vi "rx_ceEq.vi"(2 "preamble":cdb[](array[numeric])=[-0.7071067811865475+0.7071067811865476i, 0.7071067811865476+0.7071067811865475i, 0.7071067811865474-0.7071067811865477i, 0.7071067811865476+0.7071067811865475i, -0.7071067811865475+0.7071067811865476i, -0.7071067811865477-0.7071067811865475i, 0.7071067811865476+0.7071067811865475i, -0.7071067811865477-0.7071067811865475i, -0.7071067811865475+0.7071067811865476i, 0.7071067811865476+0.7071067811865475i, 0.7071067811865474-0.7071067811865477i, 0.7071067811865476+0.7071067811865475i, -0.7071067811865475+0.7071067811865476i, -0.7071067811865477-0.7071067811865475i, 0.7071067811865476+0.7071067811865475i, -0.7071067811865477-0.7071067811865475i, -0.7071067811865475+0.7071067811865476i, 0.7071067811865476+0.7071067811865475i, 0.7071067811865474-0.7071067811865477i, 0.7071067811865476+0.7071067811865475i, -0.7071067811865475+0.7071067811865476i, -0.7071067811865477-0.7071067811865475i, 0.7071067811865476+0.7071067811865475i, -0.7071067811865477-0.7071067811865475i, -0.7071067811865475+0.7071067811865476i, 0.7071067811865476+0.7071067811865475i, 0.7071067811865474-0.7071067811865477i, 0.7071067811865476+0.7071067811865475i, -0.7071067811865475+0.7071067811865476i, -0.7071067811865477-0.7071067811865475i, 0.7071067811865476+0.7071067811865475i, -0.7071067811865477-0.7071067811865475i, -0.7071067811865475+0.7071067811865476i, 0.7071067811865476+0.7071067811865475i, 0.7071067811865474-0.7071067811865477i, 0.7071067811865476+0.7071067811865475i, -0.7071067811865475+0.7071067811865476i, -0.7071067811865477-0.7071067811865475i, 0.7071067811865476+0.7071067811865475i, -0.7071067811865477-0.7071067811865475i, -0.7071067811865475+0.7071067811865476i, 0.7071067811865476+0.7071067811865475i, 0.7071067811865474-0.7071067811865477i, 0.7071067811865476+0.7071067811865475i, -0.7071067811865475+0.7071067811865476i, -0.7071067811865477-0.7071067811865475i, 0.7071067811865476+0.7071067811865475i, -0.7071067811865477-0.7071067811865475i, -0.7071067811865475+0.7071067811865476i, 0.7071067811865476+0.7071067811865475i, 0.7071067811865474-0.7071067811865477i, 0.7071067811865476+0.7071067811865475i, -0.7071067811865475+0.7071067811865476i, -0.7071067811865477-0.7071067811865475i, 0.7071067811865476+0.7071067811865475i, -0.7071067811865477-0.7071067811865475i, -0.7071067811865475+0.7071067811865476i, 0.7071067811865476+0.7071067811865475i, 0.7071067811865474-0.7071067811865477i, 0.7071067811865476+0.7071067811865475i, -0.7071067811865475+0.7071067811865476i, -0.7071067811865477-0.7071067811865475i, 0.7071067811865476+0.7071067811865475i, -0.7071067811865477-0.7071067811865475i], 3 "symbols":cdb[](array[numeric])) -> (0 "valid?":bool, 1 "eq symbols":cdb[](array[numeric]))   [LabVIEW 2014]
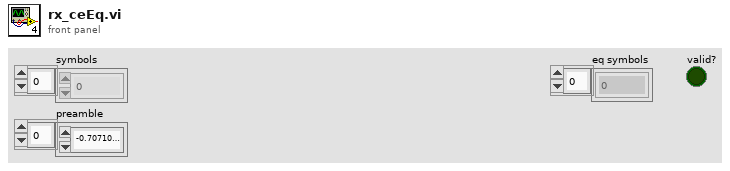
[diagram p1: front panel]
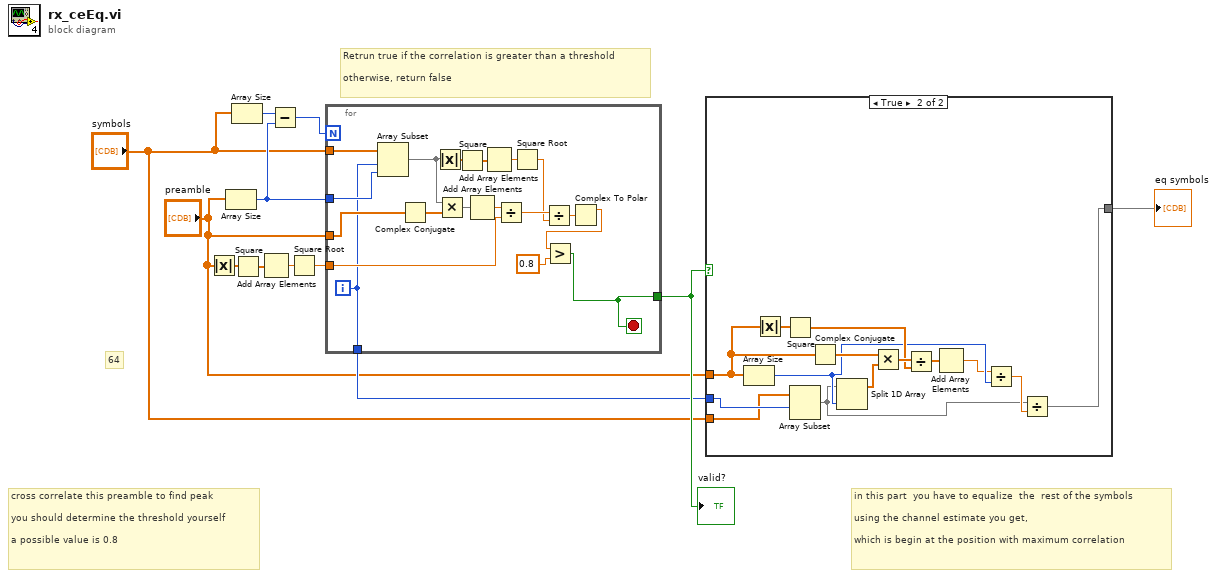
[diagram p0: block diagram]
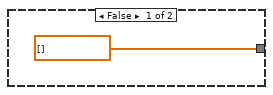
[diagram p2: hidden frame]
diagram:
  # "in this part  you have to equalize  the  rest of the symbols\n\nusing the channel estimate you get, \n\nwhich is begin at the position with maximum correlation"
  # "Retrun true if the correlation is greater than a threshold\n\notherwise, return false"
  # "cross correlate this preamble to find peak \n\nyou should determine the threshold yourself\n\na possible value is 0.8"
  # "64"
  n1 = Absolute Value(x="preamble") -> (abs(x)=w8:dbl[])
  n2 = Array Size(array="preamble") -> (size(s)=w5:i32)
  n3 = Array Size(array="symbols") -> (size(s)=w6:i32)
  n4 = Square(x=w8) -> (x^2=w11:dbl[])
  n5 = Add Array Elements(numeric array=w11) -> (sum=w10:dbl)
  n6 = Subtract(x=w6, y=w5) -> (x-y=w4:i32)
  n7 = Square Root(x=w10) -> (sqrt(x)=w9:dbl)
  n8 = for {
    N: w4 -> [_]
    tunnel: "symbols" -> [w30]
    tunnel: w5 -> [w29]
    tunnel: "preamble" -> [w23]
    tunnel: w9 -> [w21]
    tunnel: [w13] -> w7
    tunnel: [w14] -> w3
    i -> [w14]
    stop <- w13 stop-if-true
    n9 = Array Subset(array=w30, index=w14, length=w29) -> (w25:cdb[])
    n10 = Complex Conjugate(1:w23) -> (0:w24:cdb[])
    n11 = Absolute Value(x=w25) -> (abs(x)=w17:dbl[])
    n12 = Multiply(x=w25, y=w24) -> (x*y=w28:cdb[])
    n13 = Square(x=w17) -> (x^2=w27:dbl[])
    n14 = Add Array Elements(numeric array=w28) -> (sum=w22:cdb)
    n15 = Add Array Elements(numeric array=w27) -> (sum=w26:dbl)
    n16 = Divide(x=w22, y=w21) -> (x/y=w20:cdb)
    n17 = Square Root(x=w26) -> (sqrt(x)=w19:dbl)
    n18 = Divide(x=w20, y=w19) -> (x/y=w16:cdb)
    n19 = Complex To Polar(r * e^(i*theta)=w16) -> (r=w15:dbl)  [unwired: 1 out]
    n20 = Greater?(x=w15, y=0.8) -> (0:w13:bool)
  }
  "valid?" <- w7
  n21 = case shown="True" w7 {
    tunnel: [cdb[] [] w36] -> w12
    tunnel: w3 -> [_ w45]
    tunnel: "preamble" -> [_ w41]
    tunnel: "symbols" -> [_ w44]
    frame False {
    }
    frame True {
      n22 = Array Size(array=w41) -> (size(s)=w35:i32)
      n23 = Absolute Value(x=w41) -> (abs(x)=w42:dbl[])
      n24 = Square(x=w42) -> (x^2=w39:dbl[])
      n25 = Array Subset(array=w44, index=w45) -> (w32:cdb[])  [unwired: 1 in]
      n26 = Complex Conjugate(1:w41) -> (0:w43:cdb[])
      n27 = Split 1D Array(array=w32, index=w35) -> (first subarray=w37:cdb[])  [unwired: 1 out]
      n28 = Multiply(x=w43, y=w37) -> (x*y=w40:cdb[])
      n29 = Divide(x=w40, y=w39) -> (x/y=w38:cdb[])
      n30 = Add Array Elements(numeric array=w38) -> (sum=w34:cdb)
      n31 = Divide(x=w34, y=w35) -> (x/y=w33:cdb)
      n32 = Divide(x=w32, y=w33) -> (x/y=w36:cdb[])
    }
  }
  "eq symbols" <- w12
